vi "CAPTH-Flush IPC.vi"(7 "IPC In":T1) -> (8 "IPC Out":T1)   [LabVIEW 2020]
uses:
  Typedefs/CAPTH-IPC.ctl
  Typedefs/CAPTH-Start Data.ctl
  Typedefs/CAPTH-Parameters.ctl
  Typedefs/CAPTH-Stimulus.ctl
  Typedefs/CAPTH-Response.ctl
  Typedefs/CAPTH-Analysis Message.ctl
  Typedefs/CAPTH-Analysis Action.ctl
  Typedefs/CAPTH-StimCon.ctl
  Typedefs/CAPTH-Analysis Data Properties.ctl
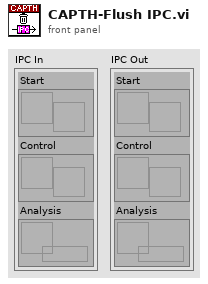
[diagram p1: front panel]
types:
  T1 = typedef "CAPTH-IPC.ctl" = cluster{"Start":refnum<notifier>, "Control":refnum<notifier>, "Analysis":refnum<queue>}
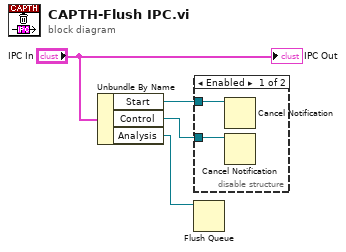
[diagram p0: block diagram]
diagram:
  n1 = Unbundle By Name("IPC In") -> ("Start"=w3:refnum<notifier>, "Control"=w2:refnum<notifier>, "Analysis"=w1:refnum<queue>)
  n2 = Flush Queue(queue=w1) -> ()  [unwired: 1 in, 3 out]
  n3 = disable-structure shown="Enabled" {
    disable-tunnel: w3 -> [w6 _]
    disable-tunnel: w2 -> [w5 _]
    frame Enabled {
      n4 = Cancel Notification(0:w6) -> ()  [unwired: 1 in, 3 out]
      n5 = Cancel Notification(0:w5) -> ()  [unwired: 1 in, 3 out]
    }
    frame Disabled {
    }
  }
  "IPC Out" <- "IPC In"
